vi "Create Random Request ID.vi"(3 "Message Loop Shift Register Data (in)":T1) -> (0 "Generated Request ID":u32, 1 "Message Loop Shift Register Data (out)":T1)   [LabVIEW 2020, in "wamplv.lvlib" / "WAMP Client.lvclass"]
uses:
  <userlib>/wamplv/WAMP Client/WAMP Client.lvclass
  <vilib>/numeric/sub_Random U32.vi
  <userlib>/wamplv/WAMP Client/WAMP Client.lvclass/WAMP Client.ctl
  <vilib>/numeric/Random Number (Range) U64.vi
  b7062e61-b09b-5842-b7d6-b9351e615acb.vi
  <userlib>/wamplv/WAMP Client/TypeDef/WAMP Error Payload.ctl
  <userlib>/wamplv/WAMP Client/TypeDef/REGISTERED or ERROR payload.ctl
  <userlib>/wamplv/WAMP Client/TypeDef/INVOCATION payload.ctl
  <userlib>/wamplv/WAMP Client/TypeDef/REGISTER Request Data.ctl
  <userlib>/wamplv/WAMP Client/TypeDef/PUBLISH Result.ctl
  <userlib>/wamplv/WAMP Client/TypeDef/PUBLISH Request Data.ctl
  <userlib>/wamplv/WAMP Client/TypeDef/Publish Requests Map.ctl
  <userlib>/wamplv/WAMP Client/TypeDef/Endpoint Data.ctl
  <userlib>/wamplv/WAMP Client/TypeDef/RESULT Payload.ctl
  <userlib>/wamplv/WAMP Client/TypeDef/CALL Request Data.ctl
  <userlib>/wamplv/WAMP Client/TypeDef/CALL Request Map.ctl
  <userlib>/wamplv/WAMP Client/TypeDef/Event Payload.ctl
  <userlib>/wamplv/WAMP Client/TypeDef/Subscribe Result.ctl
  <userlib>/wamplv/WAMP Client/TypeDef/SUBSCRIBE Request Data.ctl
  <userlib>/wamplv/WAMP Client/TypeDef/SUBSCRIBE Requests Map.ctl
  <userlib>/wamplv/WAMP Client/TypeDef/Subscription Details.ctl
  <userlib>/wamplv/WAMP Client/TypeDef/Subscriptions Map.ctl
  <userlib>/wamplv/WAMP Client/TypeDef/UNSUBSCRIBE Result.ctl
  <userlib>/wamplv/WAMP Client/TypeDef/UNSUBSCRIBE Request Data.ctl
  <userlib>/wamplv/WAMP Client/TypeDef/Unsubscribe Requests Map.ctl
  <userlib>/wamplv/WAMP Client/TypeDef/Message Loop Shift Reg Data.ctl
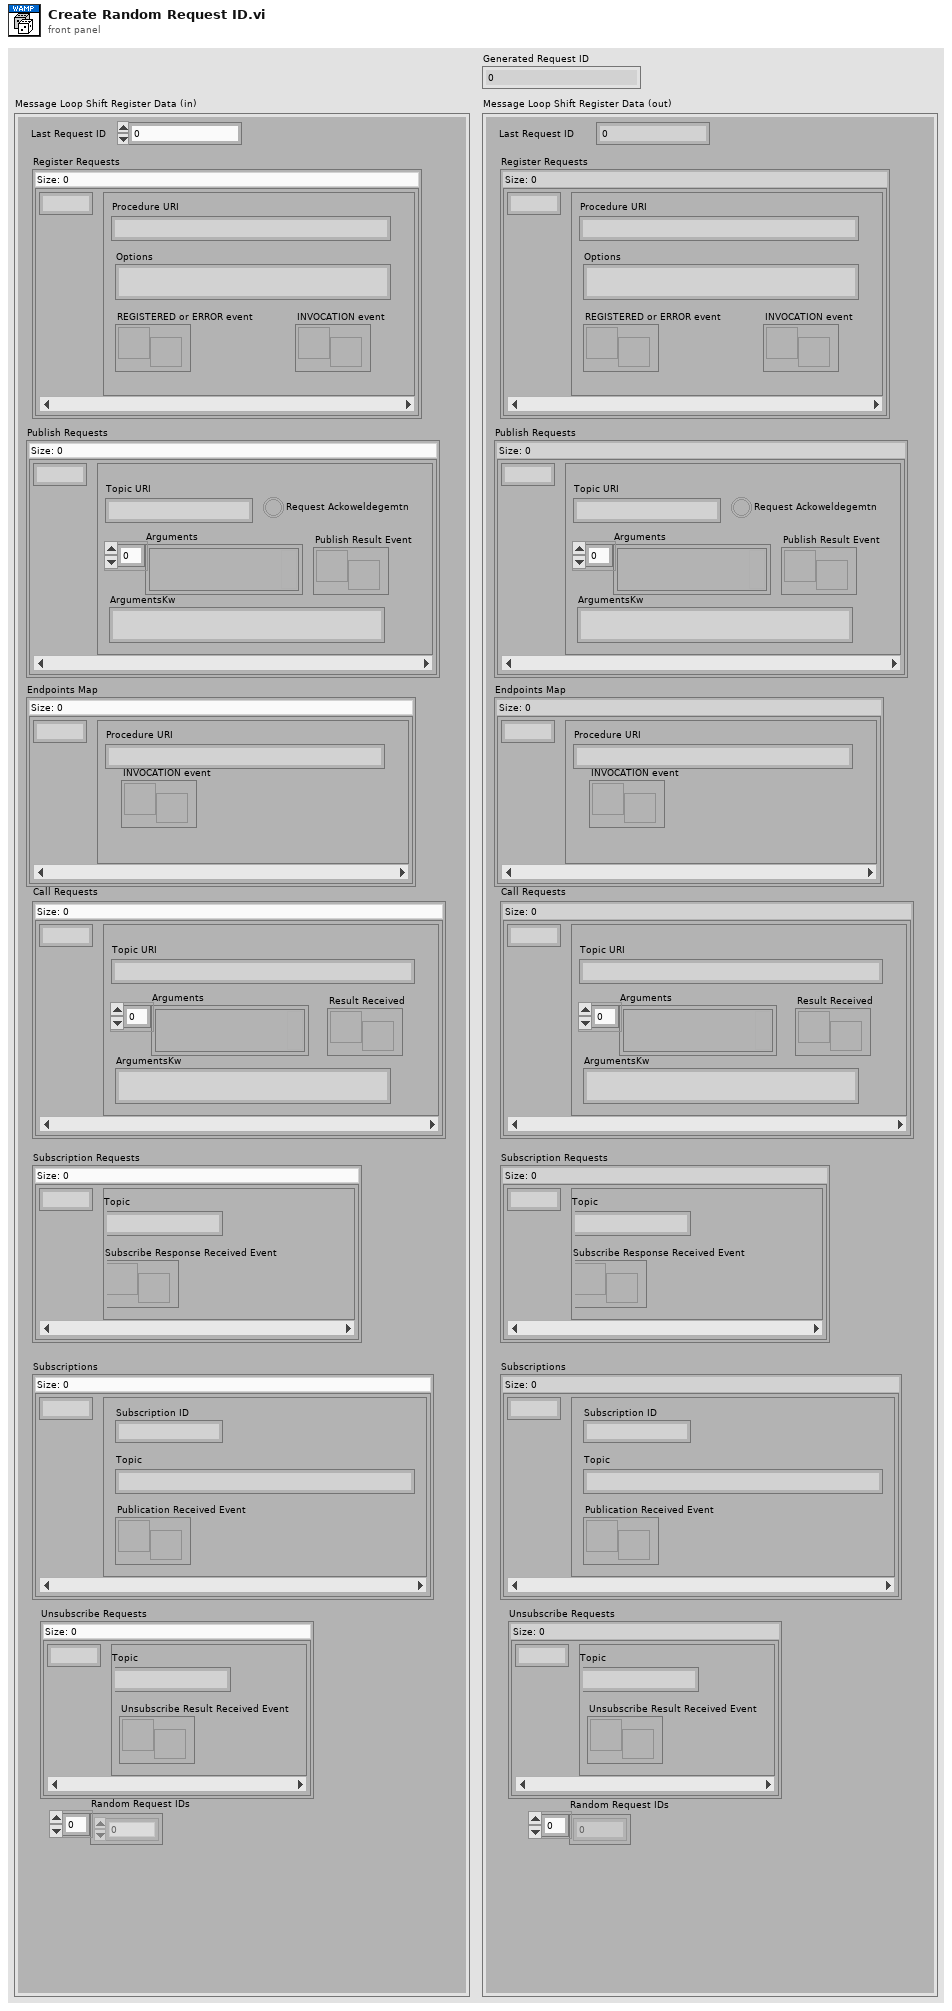
[diagram p1: front panel]
types:
  T1 = typedef "wamplv.lvlib/WAMP Client.lvclass/Message Loop Shift Reg Data.ctl" = cluster{"Last Request ID":u32, "Register Requests":map{u32, T2}, "Publish Requests":T3, "Endpoints Map":map{u32, T5}, "Call Requests":T6, "Subscription Requests":T8, "Subscriptions":T10, "Unsubscribe Requests":T12, "Random Request IDs":u32[]}
  T2 = typedef "wamplv.lvlib/WAMP Client.lvclass/REGISTER Request Data.ctl" = cluster{"Procedure URI":string, "Options":string, "REGISTERED or ERROR event":refnum<user-event>, "INVOCATION event":refnum<user-event>}
  T3 = typedef "wamplv.lvlib/WAMP Client.lvclass/Publish Requests Map.ctl" = map{u32, T4}
  T4 = typedef "wamplv.lvlib/WAMP Client.lvclass/PUBLISH Request Data.ctl" = cluster{"Topic URI":string, "Arguments":variant[], "ArgumentsKw":string, "Publish Result Event":refnum<user-event>, "Request Ackoweldegemtn":bool}
  T5 = typedef "wamplv.lvlib/WAMP Client.lvclass/Endpoint Data.ctl" = cluster{"Procedure URI":string, "INVOCATION event":refnum<user-event>}
  T6 = typedef "wamplv.lvlib/WAMP Client.lvclass/CALL Request Map.ctl" = map{u32, T7}
  T7 = typedef "wamplv.lvlib/WAMP Client.lvclass/CALL Request Data.ctl" = cluster{"Topic URI":string, "Arguments":variant[], "ArgumentsKw":string, "Result Received":refnum<user-event>}
  T8 = typedef "wamplv.lvlib/WAMP Client.lvclass/SUBSCRIBE Requests Map.ctl" = map{u32, T9}
  T9 = typedef "wamplv.lvlib/WAMP Client.lvclass/SUBSCRIBE Request Data.ctl" = cluster{"Topic":string, "Subscribe Response Received Event":refnum<user-event>}
  T10 = typedef "wamplv.lvlib/WAMP Client.lvclass/Subscriptions Map.ctl" = map{u32, T11}
  T11 = typedef "wamplv.lvlib/WAMP Client.lvclass/Subscription Details.ctl" = cluster{"Subscription ID":u32, "Topic":string, "Publication Received Event":refnum<user-event>}
  T12 = typedef "wamplv.lvlib/WAMP Client.lvclass/Unsubscribe Requests Map.ctl" = map{u32, T13}
  T13 = typedef "wamplv.lvlib/WAMP Client.lvclass/UNSUBSCRIBE Request Data.ctl" = cluster{"Topic":string, "Unsubscribe Result Received Event":refnum<user-event>}
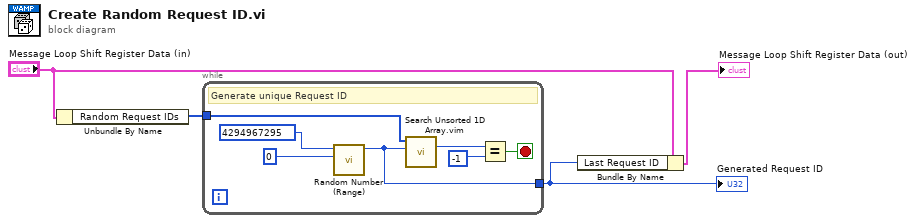
[diagram p0: block diagram]
diagram:
  n1 = Unbundle By Name("Message Loop Shift Register Data (in)") -> ("Random Request IDs"=w4:u32[])
  n2 = while {
    tunnel: w4 -> [w6]
    tunnel: [w5] -> w1
    stop <- w8 stop-if-true
    # "Generate unique Request ID"
    n3 = call-poly <vilib>:"Random Number (Range).vi"("lower bound (0)"=u32 0, "upper bound (100)"=u32 4294967295) -> ("number"=w5:u64)  [unwired: 9 in]
    n4 = call "Search Unsorted 1D Array.vim"("element"=w5, "unsorted 1D array"=w6) -> ("index of element"=w7:i32)  [unwired: 9 in]
    n5 = Equal?(x=w7, y=-1) -> (x = y?=w8:bool)
  }
  "Generated Request ID" <- w1
  n6 = Bundle By Name(cluster="Message Loop Shift Register Data (in)", "Last Request ID"=w1) -> (→"Message Loop Shift Register Data (out)":T1)
